vi "Agregar Producto a DB.vi"(8 "error in (no error)":errorcluster, 11 "Cluster":T1) -> (0 "error out":errorcluster, 3 "SUCESS?":bool)   [LabVIEW 2020, in "DataBaseSQLlite.lvlib"]
uses:
  DataBaseSQLlite.lvlib
  <vilib>/drjdpowell/SQLite Library/SQL Connection/Open (path).vi
  <vilib>/drjdpowell/SQLite Library/SQL Connection/Open (string).vi
  <vilib>/AdvancedString/Path To Command Line String.vi
  <vilib>/drjdpowell/SQLite Library/SQL Connection/Execute SQL (No results).vi
  <vilib>/drjdpowell/SQLite Library/SQL Connection/Connection.lvclass
  <vilib>/drjdpowell/SQLite Library/SQLite.lvlib
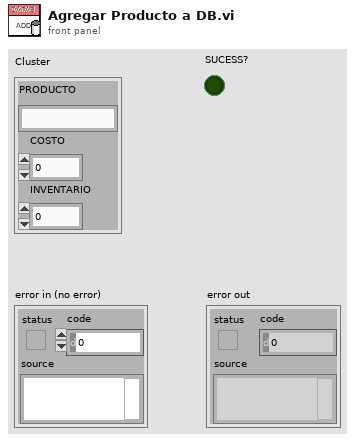
[diagram p1: front panel]
types:
  T1 = cluster{"PRODUCTO":string, "COSTO":dbl, "INVENTARIO":i64}
  T2 = typedef "ProductInvenmtarytyppedef.ctl" = cluster{"PRODUCTO":string, "COSTO":dbl, "INVENTARIO":dbl}
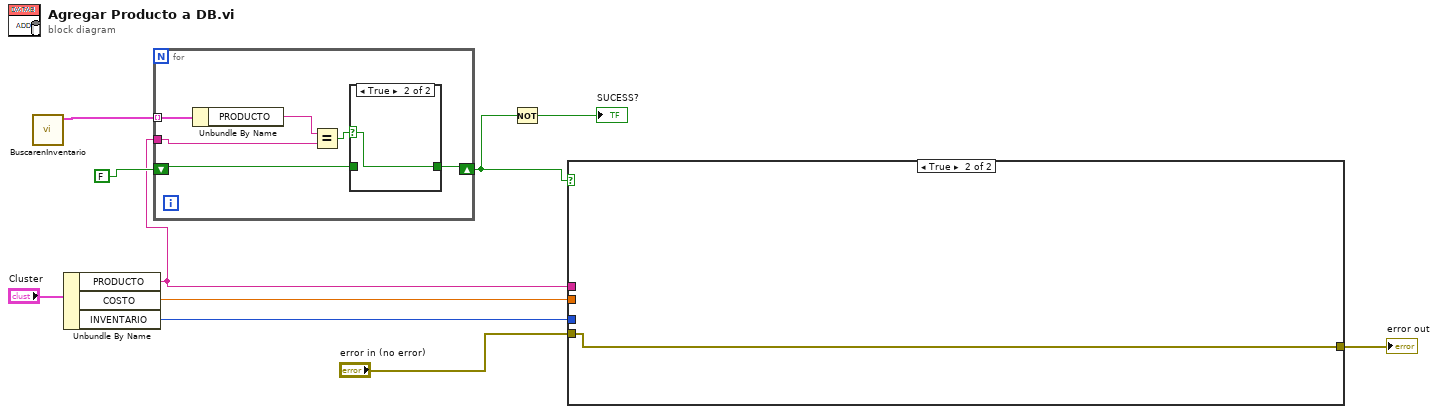
[diagram p0: block diagram]
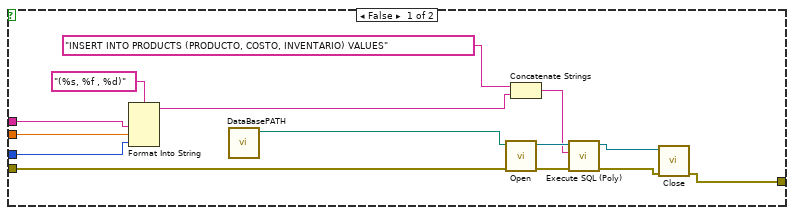
[diagram p2: hidden frame]
diagram:
  n1 = call "BuscarenInventario.vi"() -> ("Array"=w8:T2[])  [unwired: 10 in, 1 out]
  n2 = Unbundle By Name("Cluster") -> ("PRODUCTO"=w5:string, "COSTO"=w4:dbl, "INVENTARIO"=w3:i64)
  n3 = for {
    tunnel: w5 -> [w14]
    shift-right: [w12] -> w7
    shift-left: FALSE -> [w13]
    tunnel: w8 -> [w11] mode=indexing
    n4 = Unbundle By Name(w11) -> ("PRODUCTO"=w16:string)
    n5 = Equal?(x=w16, y=w14) -> (x = y?=w15:bool)
    n6 = case shown="True" w15 {
      selector: w15 -> [_ w18]
      tunnel: w13 -> [w17 _]
      tunnel: [w17 w18] -> w12
      frame False {
      }
      frame True {
      }
    }
  }
  n7 = Not(x=w7) -> (.not. x?=→"SUCESS?":bool)
  n8 = case shown="True" w7 {
    tunnel: w5 -> [w32 _]
    tunnel: w4 -> [w31 _]
    tunnel: w3 -> [w30 _]
    tunnel: "error in (no error)" -> [w23 w33]
    tunnel: [w22 w33] -> w1
    frame False {
      n9 = Format Into String(format string="(%s, %f , %d)", w32, w31, w30) -> (resulting string=w20:string)  [unwired: 2 in, 1 out]
      n10 = call "DataBasePATH.vi"() -> ("DataBase path"=w24:path)  [unwired: 11 in]
      n11 = call-poly <vilib>:"Open.vi"("error in (no error)"=w23, "db file"=w24) -> ("error out"=w27:errorcluster, "SQLite Connection"=w28:refnum<class "Connection.lvclass">)  [unwired: 8 in]
      n12 = Concatenate Strings("INSERT INTO PRODUCTS (PRODUCTO, COSTO, INVENTARIO) VALUES", w20) -> (w21:string)
      n13 = call-poly <vilib>:"Execute SQL (Poly).vi"("error in (no error)"=w27, "SQL"=w21, "SQLite Connection in"=w28) -> ("error out"=w25:errorcluster, "SQLite Connection"=w26:refnum<class "Connection.lvclass">)  [unwired: 7 in]
      n14 = call-dynamic "Close.vi"("error in (no error)"=w25, "SQLite Connection in"=w26) -> ("error out"=w22:errorcluster)  [unwired: 9 in]
    }
    frame True {
    }
  }
  "error out" <- w1
